vi "PDLM_GetLHInfo.vi"(8 "error in (no error)":errorcluster, 11 "USBIdx":i32) -> (0 "error out":errorcluster, 2 "LHInfo":T1, 3 "return type":i32)   [LabVIEW 2019]
uses:
  <userlib>/TaikoLaser/PDLM_LHInfo.ctl
  <userlib>/TaikoLaser/PDLM_DllPath_global.vi
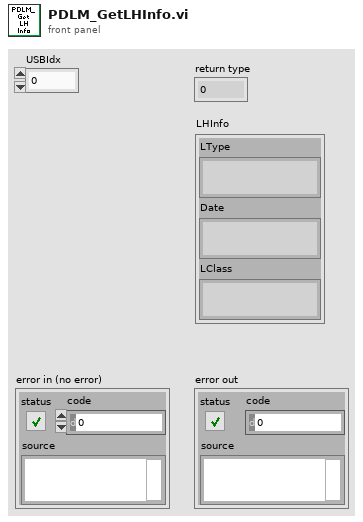
[diagram p1: front panel]
types:
  T1 = typedef "PDLM_LHInfo.ctl" = cluster{"LType":string, "Date":string, "LClass":string}
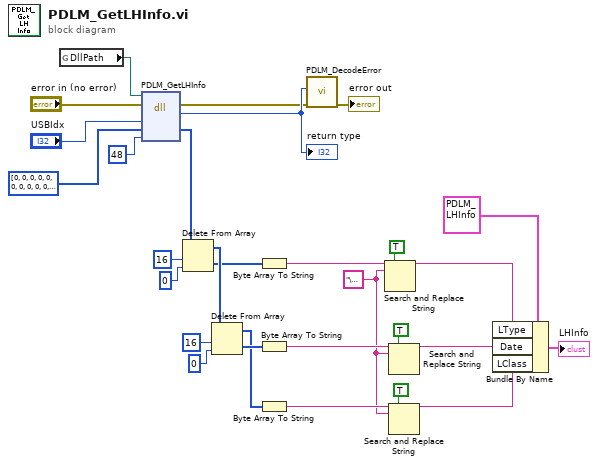
[diagram p0: block diagram]
diagram:
  w1 = "\u0000" ("search string")
  n1 = global read "PDLM_DllPath_global.vi" "DllPath"() -> (w25:path)
  n2 = dll-call lib="M:/_dev/progs/LabVIEW/_lib/PQ/Taiko/pdlm_lib.dll" fn="PDLM_GetLHInfo"(path in=w25, error in="error in (no error)", "USBIdx"="USBIdx", "Info"=u8[] [0, 0, 0, 0, 0, 0, 0, 0, 0, 0, 0, 0, 0, 0, 0, 0, 0, 0, 0, 0, 0, 0, 0, 0, 0, 0, 0, 0, 0, 0, 0, 0, 0, 0, 0, 0, 0, 0, 0, 0, 0, 0, 0, 0, 0, 0, 0, 0], "size"=u32 48) -> (error out=w27:errorcluster, "return type"=w28:i32, "Info"=w22:u8[])  [unwired: 3 in, 1 out]
  "return type" <- w28
  n3 = Delete From Array(array=w22, length=16, index=0) -> (deleted portion=w15:u8[], array with subset deleted=w17:u8[])
  n4 = Delete From Array(array=w17, length=16, index=0) -> (deleted portion=w14:u8[], array with subset deleted=w13:u8[])
  n5 = Byte Array To String(unsigned byte array=w15) -> (string=w3:string)
  n6 = Byte Array To String(unsigned byte array=w14) -> (string=w8:string)
  n7 = Byte Array To String(unsigned byte array=w13) -> (string=w6:string)
  n8 = call <userlib>:"PDLM_DecodeError.vi"("error in (no error)"=w27, "code"=w28) -> ("error out"=→"error out":errorcluster)  [unwired: 7 in, 2 out]
  n9 = Search and Replace String(replace all?=TRUE ("replace all? (F)"), input string=w3, search string=w1) -> (result string=w2:string)  [unwired: 5 in, 3 out]
  n10 = Search and Replace String(replace all?=TRUE ("replace all? (F)"), input string=w8, search string=w1) -> (result string=w7:string)  [unwired: 5 in, 3 out]
  n11 = Search and Replace String(replace all?=TRUE ("replace all? (F)"), input string=w6, search string=w1) -> (result string=w5:string)  [unwired: 5 in, 3 out]
  n12 = Bundle By Name(cluster=T1 {"LType"="\u0000\u0000\u0000\u0000\u0000\u0000\u0000\u0000\u0000\u0000\u0000\u0000\u0000\u0000\u0000\u0000", "Date"="\u0000\u0000\u0000\u0000\u0000\u0000\u0000\u0000\u0000\u0000\u0000\u0000\u0000\u0000\u0000\u0000", "LClass"="\u0000\u0000\u0000\u0000\u0000\u0000\u0000\u0000\u0000\u0000\u0000\u0000\u0000\u0000\u0000\u0000"} ("LHInfo"), "LType"=w2, "Date"=w7, "LClass"=w5) -> (→"LHInfo":T1)
